vi "Do.vi"(8 "error in (no error)":errorcluster, 10 "Actor in":refnum<class "Actor.lvclass">, 11 "AFG Report Event Msg":refnum<class "AFG Report Event Msg.lvclass">) -> (0 "error out":errorcluster, 2 "Actor out":refnum<class "Actor.lvclass">)   [LabVIEW 2020, in "Actor_AFG.lvlib" / "AFG Report Event Msg.lvclass"]
doc: "This VI delivers the message to the actor by calling the appropriate method(s) on the actor."
uses:
  AFG Report Event Msg.lvclass
  <vilib>/ActorFramework/Actor/Actor.lvclass
  AFG Report Event Msg.lvclass/AFG Report Event Msg.ctl
  I_AFG/I_AFG.lvclass
  9b391c87-dee2-48ea-81da-579391dd1fe1.vi
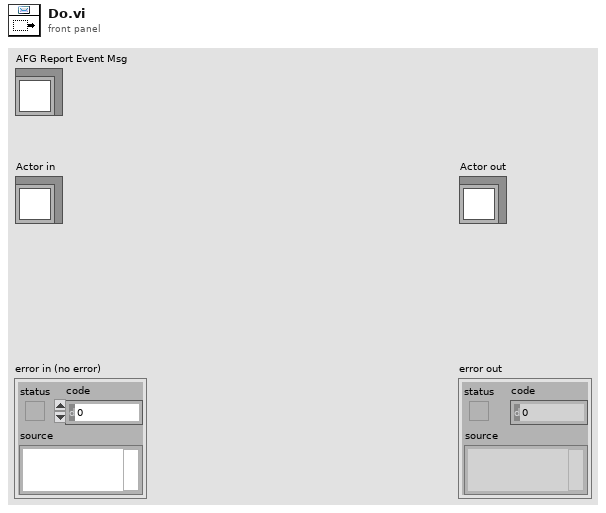
[diagram p1: front panel]
types:
  T1 = typedef "Actor_AFG.lvlib/Actor_AFG.lvclass/AFG_Event.ctl" = enum16{"General Event", "Inited", "Output", "Waveform Set", "Error"}
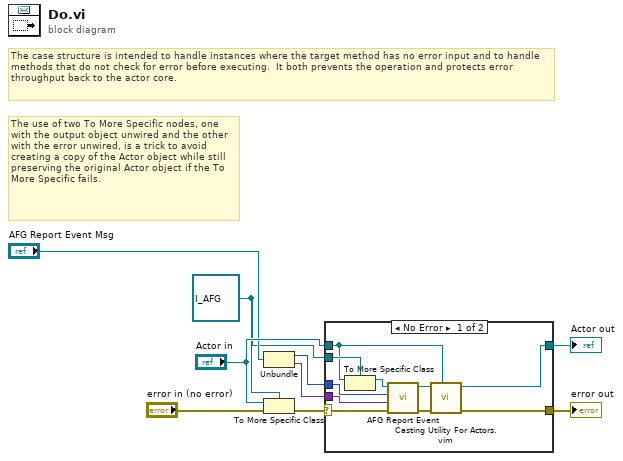
[diagram p0: block diagram]
diagram:
  w4 = refnum<class "I_AFG.lvclass"> refnum ("Actor in")
  # "The use of two To More Specific nodes, one with the output object unwired and the other with the error unwired, is a trick to avoid creating a copy of the Actor object while still preserving the original Actor object if the To More Specific fails."
  # "The case structure is intended to handle instances where the target method has no error input and to handle methods that do not check for error before executing.  It both prevents the operation and protects error throughput back to the actor core."
  n1 = Unbundle("AFG Report Event Msg") -> (w2:T1, w1:variant)
  n2 = To More Specific Class(target class=w4, reference="Actor in", error in="error in (no error)") -> (error out=w3:errorcluster)  [unwired: 1 out]
  n3 = case shown="No Error" w3 {
    selector: w3 -> [w19 w21]
    tunnel: [w13 w21] -> w9
    tunnel: [w14 w20] -> w8
    tunnel: "Actor in" -> [w16 w20]
    tunnel: w4 -> [w17 _]
    tunnel: w2 -> [w11 _]
    tunnel: w1 -> [w10 _]
    frame No Error {
      n4 = To More Specific Class(target class=w17, reference=w16) -> (specific class reference=w18:refnum<class "I_AFG.lvclass">)  [unwired: 1 in, 1 out]
      n5 = call-dynamic "AFG Report Event.vi"("error in (no error)"=w19, "Event Data"=w10, "Report Events"=w11, "I_AFG in"=w18) -> ("error out"=w12:errorcluster, "I_AFG out"=w15:refnum<class "I_AFG.lvclass">)  [unwired: 6 in]
      n6 = call "Casting Utility For Actors.vim"("type"=w16, "error in (no error)"=w12, "Actor in"=w15) -> ("error out"=w13:errorcluster, "Actor out"=w14:refnum<class "Actor.lvclass">)  [unwired: 7 in]
    }
    frame Error {
      # "If type check fails, pass the original object out again."
    }
  }
  "error out" <- w9
  "Actor out" <- w8
